vi "Synchronous Dialog.vi"(4 "Python Message ID":i32, 5 "Script ID":i64, 7 "Server Alias":string, 8 "Error In":errorcluster, 10 "Send Response":bool, 11 "Message In":string) -> (0 "Error Out":errorcluster)   [LabVIEW 2013]
doc: "This is an example of a dialog box for TestScript. The Python side can tell this dialog to run, asking for user input."
uses:
  LabVIEW Core/TS.lvlib
panel:
  out "Message Indicator":string
  in  "OK":bool
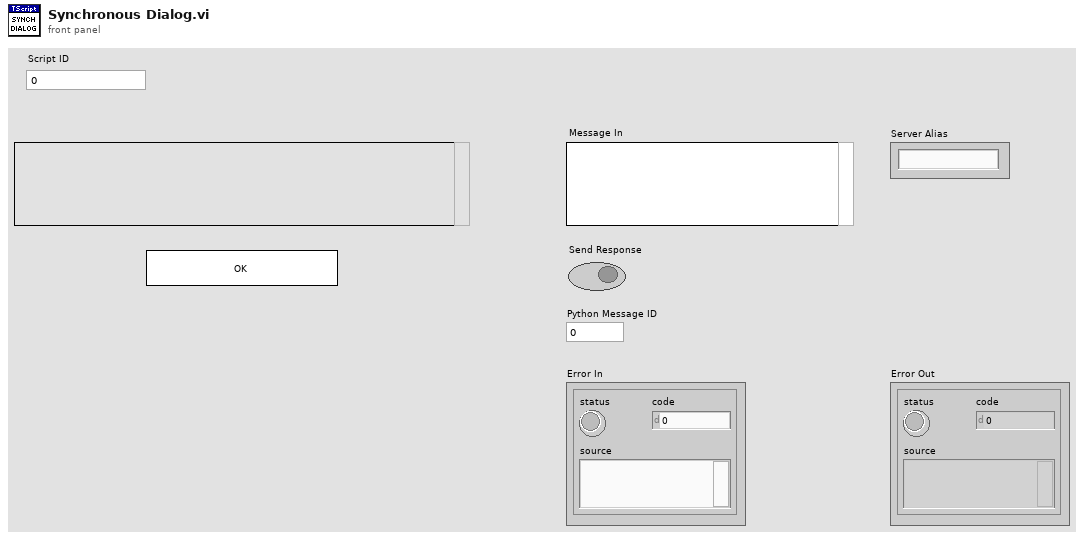
[diagram p1: front panel]
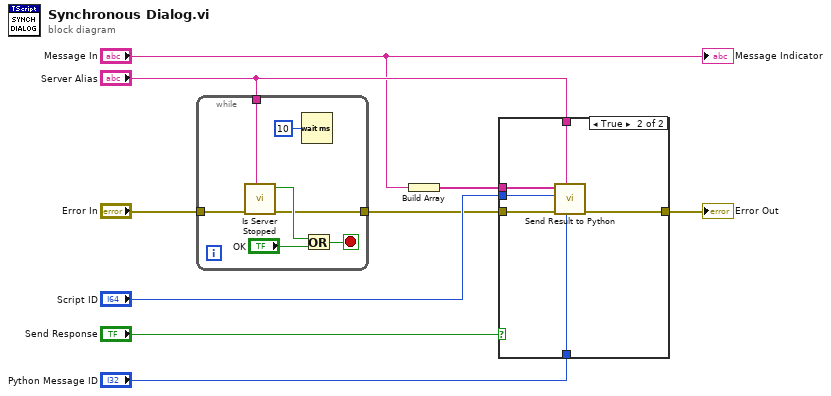
[diagram p0: block diagram]
diagram:
  n1 = while {
    tunnel: "Server Alias" -> [w12]
    tunnel: "Error In" -> [w11]
    tunnel: [w10] -> w4
    stop <- w14 stop-if-true
    n2 = call "Is Server Stopped.vi"("Server Alias"=w12, "Error In"=w11) -> ("Error Out"=w10:errorcluster, "Server Stopped"=w13:bool)  [unwired: 8 in]
    n3 = Wait (ms)(milliseconds to wait=u32 10) -> ()  [unwired: 1 out]
    n4 = Or(x=w13, y="OK") -> (x .or. y?=w14:bool)
  }
  n5 = Build Array("Message In") -> (w9:string[])
  n6 = case shown="True" "Send Response" {
    tunnel: w9 -> [_ w23]
    tunnel: "Script ID" -> [_ w22]
    tunnel: "Python Message ID" -> [_ w21]
    tunnel: w4 -> [w17 w20]
    tunnel: [w17 w19] -> w3
    tunnel: "Server Alias" -> [_ w18]
    frame False {
    }
    frame True {
      n7 = call "Send Result to Python.vi"("Python Message ID"=w21, "Server Alias"=w18, "error in (no error)"=w20, "Script ID"=w22, "Result Data"=w23) -> ("error out"=w19:errorcluster)  [unwired: 6 in]
    }
  }
  "Error Out" <- w3
  "Message Indicator" <- "Message In"
